vi "Global-trigger-test.vi"(8 "Boolean 2":bool) -> ()   [LabVIEW 2020]
panel:
  out "Boolean":bool
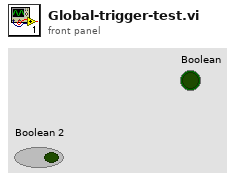
[diagram p1: front panel]
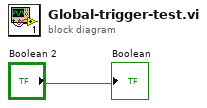
[diagram p0: block diagram]
diagram:
  "Boolean" <- "Boolean 2"
